vi "rqp_Start Session.vi"(4 "Show in Debugger?":bool=TRUE, 6 "Message Priority":T1=enum."Normal", 7 "Caller in":refnum<class "Worker.lvclass">, 8 "error in":errorcluster, 10 "Data in":T2, 11 "Pumps Worker in":refnum<class "Pumps Worker.lvclass">) -> (0 "error out":errorcluster, 3 "dup Pumps Worker out":refnum<class "Pumps Worker.lvclass">, 5 "dup Caller out":refnum<class "Worker.lvclass">)   [LabVIEW 2023, in "pump_Lib.lvlib" / "Pumps Worker.lvclass"]
doc: "This VI sends a <b>Public API Request</b> message to an MHL case of the Worker that owns this VI.\n---\nWorkers Public API Request Case"
uses:
  Pumps Worker.lvclass
  C:/Program Files/National Instruments/LabVIEW 2023/vi.lib/addons/_Workers/Library/Classes/Worker/Worker.lvclass
  <vilib>/addons/_Workers/Library/Classes/Worker/Worker.lvclass
  rqp_Start Session.ctl
  <vilib>/addons/_Workers/Library/Classes/Message/Priority.ctl
  <vilib>/addons/_Workers/Library/Case Label.ctl
  <vilib>/addons/_Workers/Library/Classes/Message Queue/Message Queue.lvclass
  <vilib>/addons/_Workers/Library/Workers.lvlib
  <vilib>/addons/_Workers/Library/Classes/Message/Message.lvclass
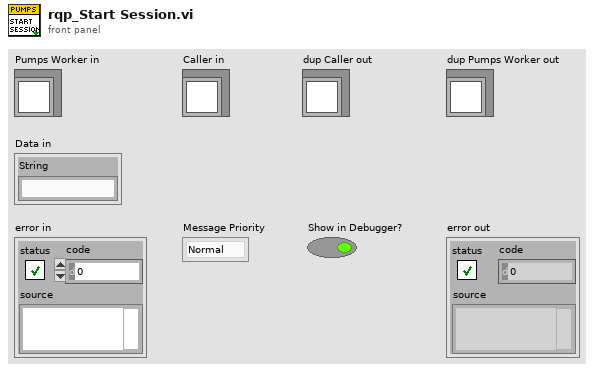
[diagram p1: front panel]
types:
  T1 = typedef "Workers.lvlib/Message.lvclass/Priority.ctl" = enum16{"Low", "Normal", "High"}
  T2 = typedef "pump_Lib.lvlib/Pumps Worker.lvclass/rqp_Start Session.ctl" = cluster{"String":string}
  T3 = typedef "Workers.lvlib/Case Label.ctl" = string
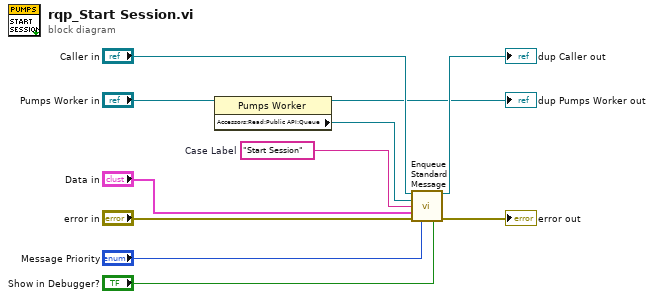
[diagram p0: block diagram]
diagram:
  w1 = T3 "Start Session"  # Case Label
  n1 = property class="Pumps Worker"(reference="Pumps Worker in") -> (reference out=→"dup Pumps Worker out":refnum<class "Pumps Worker.lvclass">, "Accessors:Read:Public API:Queue"=w2:refnum<class "Message Queue.lvclass">)  [unwired: 1 in, 1 out]
  n2 = call-dynamic "Enqueue Standard Message.vi"("Worker"="Caller in", "Message Queue"=w2, "Case Label"=w1, "Data"="Data in", "error in (no error)"="error in", "Priority (Normal)"="Message Priority", "Send Message to Debugger? (T)"="Show in Debugger?") -> ("dup Worker out"=→"dup Caller out":refnum<class "Worker.lvclass">, "error out"=→"error out":errorcluster)  [unwired: 7 in]
